vi "Introspection Core.vi"(8 "error in (no error)":errorcluster, 11 "CS++DSCAlarmViewer in":refnum<class "CS++DSCAlarmViewer.lvclass">) -> (0 "error out":errorcluster, 2 "CS++Messages":refnum<class "Message.lvclass">[](array[class]), 3 "CS++DSCAlarmViewer out":refnum<class "CS++DSCAlarmViewer.lvclass">)   [LabVIEW 2014, in "CS++DSCAlarmViewer.lvlib" / "CS++DSCAlarmViewer.lvclass"]
doc: "This vi delivers a list with all messages this actor reacts to. \n\nNote that all inherited classes have to overwrite it."
uses:
  CS++DSCAlarmViewer.lvclass
  <vilib>/ActorFramework/Message/Message.lvclass
  CSPP_Core/Actors/CS++GUIActor/CS++GUIActor.lvclass
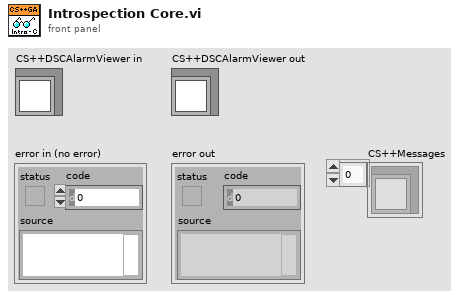
[diagram p1: front panel]
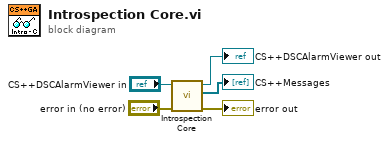
[diagram p0: block diagram]
diagram:
  n1 = call-parent "Introspection Core.vi"("error in (no error)"="error in (no error)", "CS++GUIActor in"="CS++DSCAlarmViewer in") -> ("error out"=→"error out":errorcluster, "CS++Messages"=→"CS++Messages":refnum<class "Message.lvclass">[], "CS++GUIActor out"=→"CS++DSCAlarmViewer out":refnum<class "CS++DSCAlarmViewer.lvclass">)  [unwired: 7 in]
